vi "Destroy DCPower session.vi"(6 "Session manager service gRPC ID":T4, 7 "Discovery service gRPC ID":T4, 8 "error in":errorcluster, 10 "sessions":T1[](array[typedef]), 11 "Instrument handles":refnum<k15>[](array[refnum])) -> (0 "error out":errorcluster)   [LabVIEW 2020, in "NIDCPowerSourceDCVoltage.lvlib"]
uses:
  NIDCPowerSourceDCVoltage.lvlib
  <vilib>/gRPC/LabVIEW gRPC Library/Shared/grpcId.ctl
  <vilib>/MeasurementLink/MeasurementLink Session Management Client/RPC Messages/ni_measurementlink_sessionmanagement_v1_SessionInformation.ctl
  <vilib>/MeasurementLink/MeasurementLink Session Management Client/RPC Messages/nidevice_grpc_Session.ctl
  <vilib>/MeasurementLink/MeasurementLink Session Management Client/RPC Messages/ni_measurementlink_sessionmanagement_v1_ChannelMapping.ctl
  <vilib>/MeasurementLink/MeasurementLink Session Management Client/RPC Messages/ni_measurementlink_sessionmanagement_v1_UnreserveSessionsRequest.ctl
  <vilib>/MeasurementLink/MeasurementLink Discovery Client/MeasurementLink Discovery Client.lvlib
  <vilib>/MeasurementLink/MeasurementLink Session Management Client/MeasurementLink Session Management Client.lvlib
  <vilib>/gRPC/LabVIEW gRPC Library/grpc-lvsupport-release.lvlib
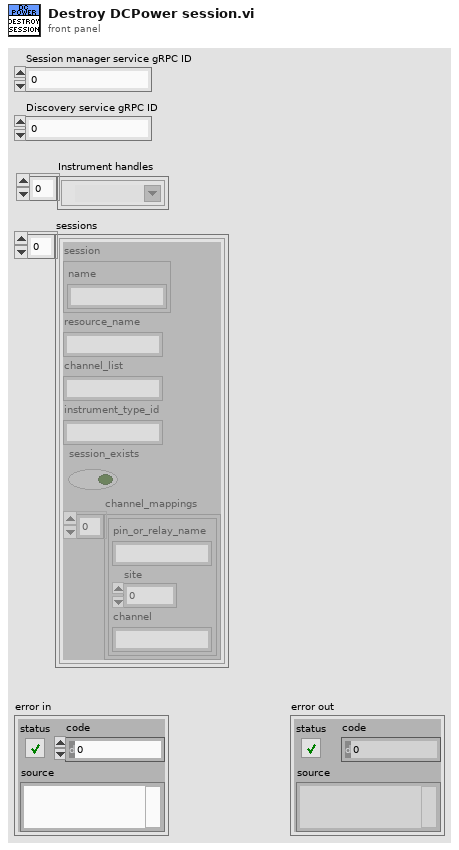
[diagram p1: front panel]
types:
  T1 = typedef "MeasurementLink Session Management Client.lvlib/ni_measurementlink_sessionmanagement_v1_SessionInformation.ctl" = cluster{"session":T2, "resource_name":string, "channel_list":string, "instrument_type_id":string, "session_exists":bool, "channel_mappings":T3[]}
  T2 = typedef "MeasurementLink Session Management Client.lvlib/nidevice_grpc_Session.ctl" = cluster{"name":string}
  T3 = typedef "MeasurementLink Session Management Client.lvlib/ni_measurementlink_sessionmanagement_v1_ChannelMapping.ctl" = cluster{"pin_or_relay_name":string, "site":i32, "channel":string}
  T4 = typedef "grpc-lvsupport-release.lvlib/grpcId.ctl" = u64
  T5 = typedef "MeasurementLink Session Management Client.lvlib/ni_measurementlink_sessionmanagement_v1_UnreserveSessionsRequest.ctl" = cluster{"sessions":T1[]}
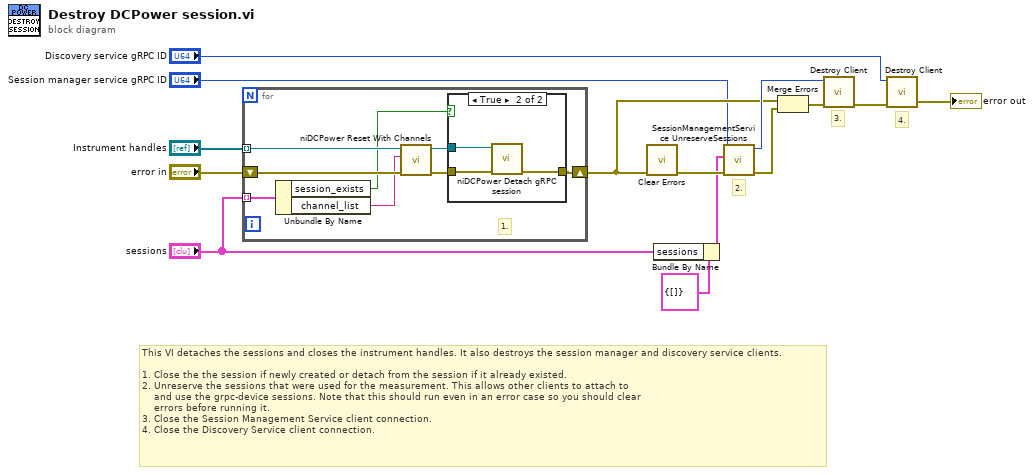
[diagram p0: block diagram]
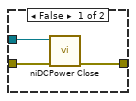
[diagram p2: hidden frame]
diagram:
  # "This VI detaches the sessions and closes the instrument handles. It also destroys the session manager and discovery service clients.\n\n1. Close the the session if newly created or detach from the session if it already existed.\n2. Unreserve the sessions that were used for the measurement. This allows other clients to attach to\n    and use the grpc-device sessions. Note that this should run even in an error case so you should clear \n    errors before running it.\n3. Close the Session Management Service client connection.\n4. Close the Discovery Service client connection."
  # "2."
  # "4."
  # "3."
  n1 = for {
    tunnel: "Instrument handles" -> [w22] mode=indexing
    shift-right: [w18] -> w5
    shift-left: "error in" -> [w21]
    tunnel: "sessions" -> [w17] mode=indexing
    # "1."
    n2 = Unbundle By Name(w17) -> ("session_exists"=w15:bool, "channel_list"=w16:string)
    n3 = call <instrlib>:"niDCPower Reset With Channels.vi"("error in (no error)"=w21, "channel name"=w16, "instrument handle"=w22) -> ("error out"=w20:errorcluster, "instrument handle out"=w19:refnum<k15>)  [unwired: 7 in]
    n4 = case shown="True" w15 {
      tunnel: w19 -> [w25 w26]
      tunnel: w20 -> [w24 w27]
      tunnel: [w23 w28] -> w18
      frame False {
        n5 = call <instrlib>:"niDCPower Close.vi"("error in (no error)"=w24, "instrument handle"=w25) -> ("error out"=w23:errorcluster)  [unwired: 9 out]
      }
      frame True {
        n6 = call <instrlib>:"niDCPower Detach gRPC session.vi"("error in (no error)"=w27, "instrument handle"=w26) -> ("error out"=w28:errorcluster)  [unwired: 9 in]
      }
    }
  }
  n7 = call <vilib>:"Clear Errors.vi"("error in (no error)"=w5) -> ("error out"=w11:errorcluster)  [unwired: 5 in, 1 out]
  n8 = Bundle By Name(cluster=T5 {"sessions"=[]} ("Request Data"), "sessions"="sessions") -> (w9:T5)
  n9 = call <vilib>:"SessionManagementService UnreserveSessions.vi"("error in"=w11, "Request Data"=w9, "gRPC ID"="Session manager service gRPC ID") -> ("error out"=w7:errorcluster, "gRPC ID out"=w13:T4)  [unwired: 6 in, 1 out]
  n10 = Merge Errors(w5, w7) -> (w8:errorcluster)
  n11 = call <vilib>:"Destroy Client.vi"("error in"=w8, "gRPC ID"=w13) -> ("error out"=w12:errorcluster)  [unwired: 9 in]
  n12 = call <vilib>:"Destroy Client.vi"("error in"=w12, "gRPC ID"="Discovery service gRPC ID") -> ("error out"=→"error out":errorcluster)  [unwired: 9 in]
